vi "Radians To Degrees.vi"(11 "Degrees":dbl) -> (3 "Radians":dbl)   [LabVIEW 2015]
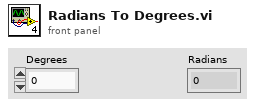
[diagram p1: front panel]
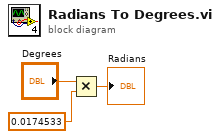
[diagram p0: block diagram]
diagram:
  n1 = Multiply(x="Degrees", y=0.0174533) -> (x*y=→"Radians":dbl)
